vi "SetPortsAndSpeedsGain.vi"(9 "Ports and Speeds":refnum<vi>, 10 "SpeedTable":refnum<k24>, 11 "ComboBox in":refnum<vi>) -> ()   [LabVIEW 2019]
uses:
  Dependencies/PVCamNET.dll
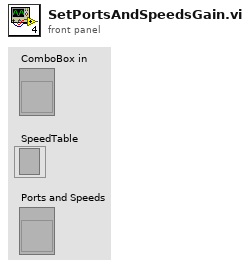
[diagram p1: front panel]
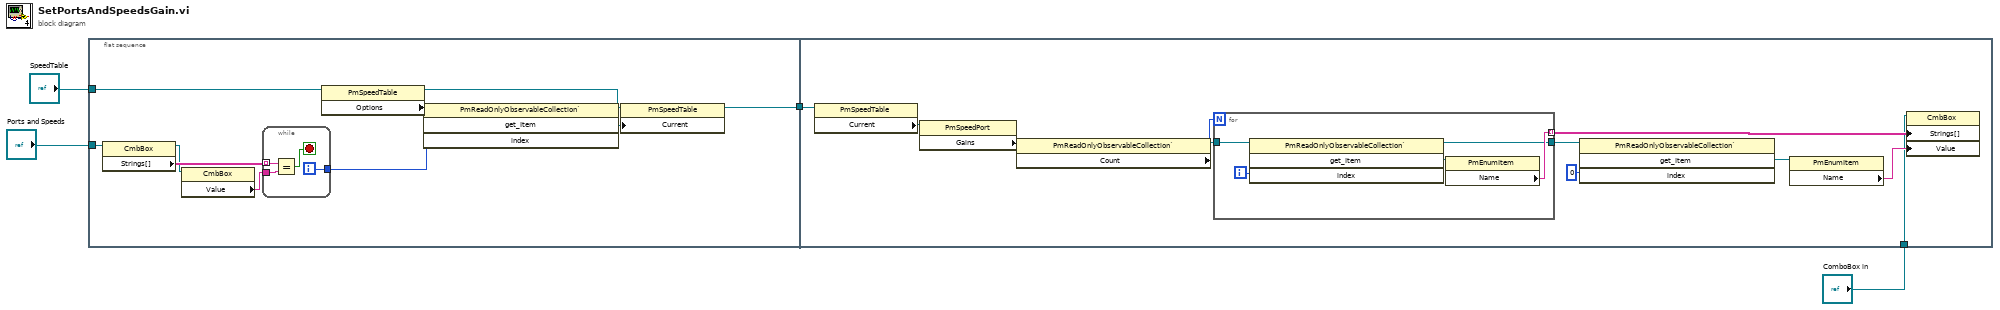
[diagram p0: block diagram]
diagram:
  n1 = flat-sequence {
    tunnel: "SpeedTable" -> [w9]
    tunnel: [w8] -> w4
    tunnel: "Ports and Speeds" -> [w5]
    tunnel: w4 -> [w29]
    tunnel: "ComboBox in" -> [w19]
    frame #0 {
      n2 = property class="CmbBox"(reference=w5) -> (reference out=w7:refnum<vi>, "Strings[]"=w14:string[])  [unwired: 1 in, 1 out]
      n3 = property class="CmbBox"(reference=w7) -> ("Value"=w6:string)  [unwired: 1 in, 2 out]
      n4 = while {
        tunnel: w14 -> [w18] mode=indexing
        tunnel: [w16] -> w13
        tunnel: w6 -> [w15]
        i -> [w16]
        stop <- w17 stop-if-true
        n5 = Equal?(x=w18, y=w15) -> (x = y?=w17:bool)
      }
      n6 = property class="PmSpeedTable"(reference=w9) -> (reference out=w11:refnum<k24>, "Options"=w10:refnum<k24>)  [unwired: 1 in, 1 out]
      n7 = invoke class="PmReadOnlyObservableCollection`" method="get_Item"(reference=w10, "index"=w13) -> ("get_Item"=w12:refnum<k24>)  [unwired: 2 in, 3 out]
      n8 = property class="PmSpeedTable"(reference=w11, "Current"=w12) -> (reference out=w8:refnum<k24>)  [unwired: 1 in, 1 out]
    }
    frame #1 {
      n9 = property class="PmSpeedTable"(reference=w29) -> ("Current"=w28:refnum<k24>)  [unwired: 1 in, 2 out]
      n10 = property class="PmSpeedPort"(reference=w28) -> ("Gains"=w27:refnum<k24>)  [unwired: 1 in, 2 out]
      n11 = property class="PmReadOnlyObservableCollection`"(reference=w27) -> (reference out=w25:refnum<k24>, "Count"=w26:i32)  [unwired: 1 in, 1 out]
      n12 = for {
        N: w26 -> [_]
        tunnel: w25 -> [w34]
        tunnel: [w31] -> w24 mode=indexing
        tunnel: [w30] -> w23
        i -> [w33]
        n13 = invoke class="PmReadOnlyObservableCollection`" method="get_Item"(reference=w34, "index"=w33) -> (reference out=w30:refnum<k24>, "get_Item"=w32:refnum<k24>)  [unwired: 2 in, 2 out]
        n14 = property class="PmEnumItem"(reference=w32) -> ("Name"=w31:string)  [unwired: 1 in, 2 out]
      }
      n15 = invoke class="PmReadOnlyObservableCollection`" method="get_Item"(reference=w23, "index"=0) -> ("get_Item"=w21:refnum<k24>)  [unwired: 2 in, 3 out]
      n16 = property class="PmEnumItem"(reference=w21) -> ("Name"=w20:string)  [unwired: 1 in, 2 out]
      n17 = property class="CmbBox"(reference=w19, "Strings[]"=w24, "Value"=w20) -> ()  [unwired: 1 in, 2 out]
    }
  }
